vi "Write message of the file header.vi"(8 "error in (no error)":errorcluster, 10 "message of the file header":string="----------------\nLOG FILE OF ACS\n----------------\n\nThis is the log file of ACS.  In this file, the messages generated during the execution of the softrware,\nas well as the commands received from the Graphical User Interface of SPARC4 are logged. ", 11 "Log File in":refnum<class "CCS_Log File.lvclass">) -> (0 "error out":errorcluster, 3 "Log File out":refnum<class "CCS_Log File.lvclass">)   [LabVIEW 2018, in "CCS_Log File.lvclass"]
uses:
  CCS_Log File.lvclass
  CCS_Log File.lvclass/CCS_Log File.ctl
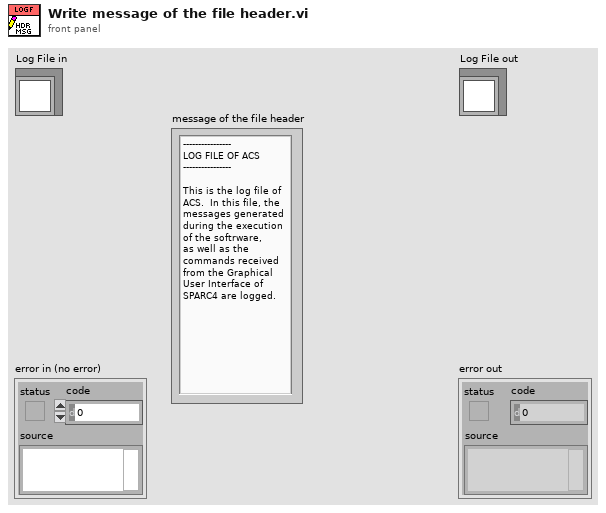
[diagram p1: front panel]
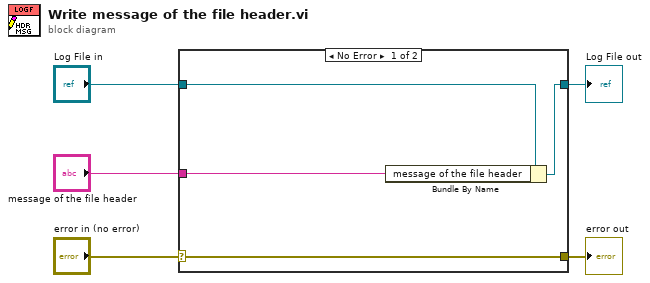
[diagram p0: block diagram]
diagram:
  n1 = case shown="No Error" "error in (no error)" {
    selector: "error in (no error)" -> [w9 w10]
    tunnel: [w9 w10] -> w4
    tunnel: [w7 w11] -> w2
    tunnel: "Log File in" -> [w8 w11]
    tunnel: "message of the file header" -> [w6 _]
    frame No Error {
      n2 = Bundle By Name(cluster=w8, "message of the file header"=w6) -> (w7:refnum<class "CCS_Log File.lvclass">)
    }
    frame Error {
    }
  }
  "error out" <- w4
  "Log File out" <- w2
